vi "saveClampResults-v03.vi"(0 "controls array":refnum<vi>[](array[refnum]), 1 "protocol or memtest":enum16{"protocol", "memtest", "dual"}(ring), 2 "ExpPhase":string, 3 "which clamp":enum16{"VClamp", "IClamp"}(ring), 5 "view profile":waveform(dbl)[](array[waveform]), 9 "rec profile":waveform(dbl)[](array[waveform]), 11 "error in":errorcluster caption="error in (no error)", 12 "metadata to save":T1 {"cell stats"."STD" format="%010.2f"; "cell stats"."Variance" format="%010.2f"; "cell stats"."Rt (MOhms)" format="%010.2f"; "cell stats"."tau (ms)" format="%08.2g"; "cell stats"."Cm (pF)" format="%08.2f"; "cell stats"."Ra (MOhms)" format="%010.2f"; "cell stats"."Rm (MOhms)" format="%010.2f"; "cell stats"."Ihold (pA)" format="%010.2f"}, 14 "Save to (folder dir)":path=path "C:/DATA/8-27-15 save func testing") -> (4 "controls array out":refnum<vi>[](array[refnum]), 15 "error out":errorcluster)   [LabVIEW 2019]
uses:
  autoWC/get_data_from_control_boolean.vi
  wc_protocol_v1.003 Folder/whole_cell_protocol/Controls/cell_stats-v02.ctl
  wc_protocol_v1.003 Folder/whole_cell_protocol/Controls/metadata_to_save.ctl
panel:
  out "rec path out":path
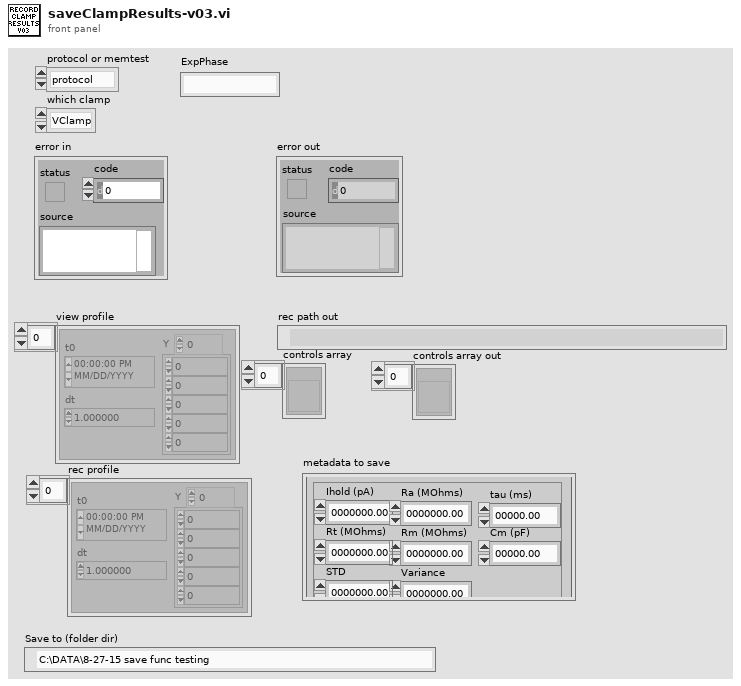
[diagram p1: front panel]
types:
  T1 = typedef "metadata_to_save.ctl" = cluster{"cell stats":T2}
  T2 = typedef "cell_stats-v02.ctl" = cluster{"Ihold (pA)":dbl, "Rm (MOhms)":dbl, "Ra (MOhms)":dbl, "Cm (pF)":dbl, "tau (ms)":dbl, "Rt (MOhms)":dbl, "Variance":dbl, "STD":dbl}
  T3 = enum16{"open", "replace", "create", "open or create", "replace or create", "replace or create with confirmation"}
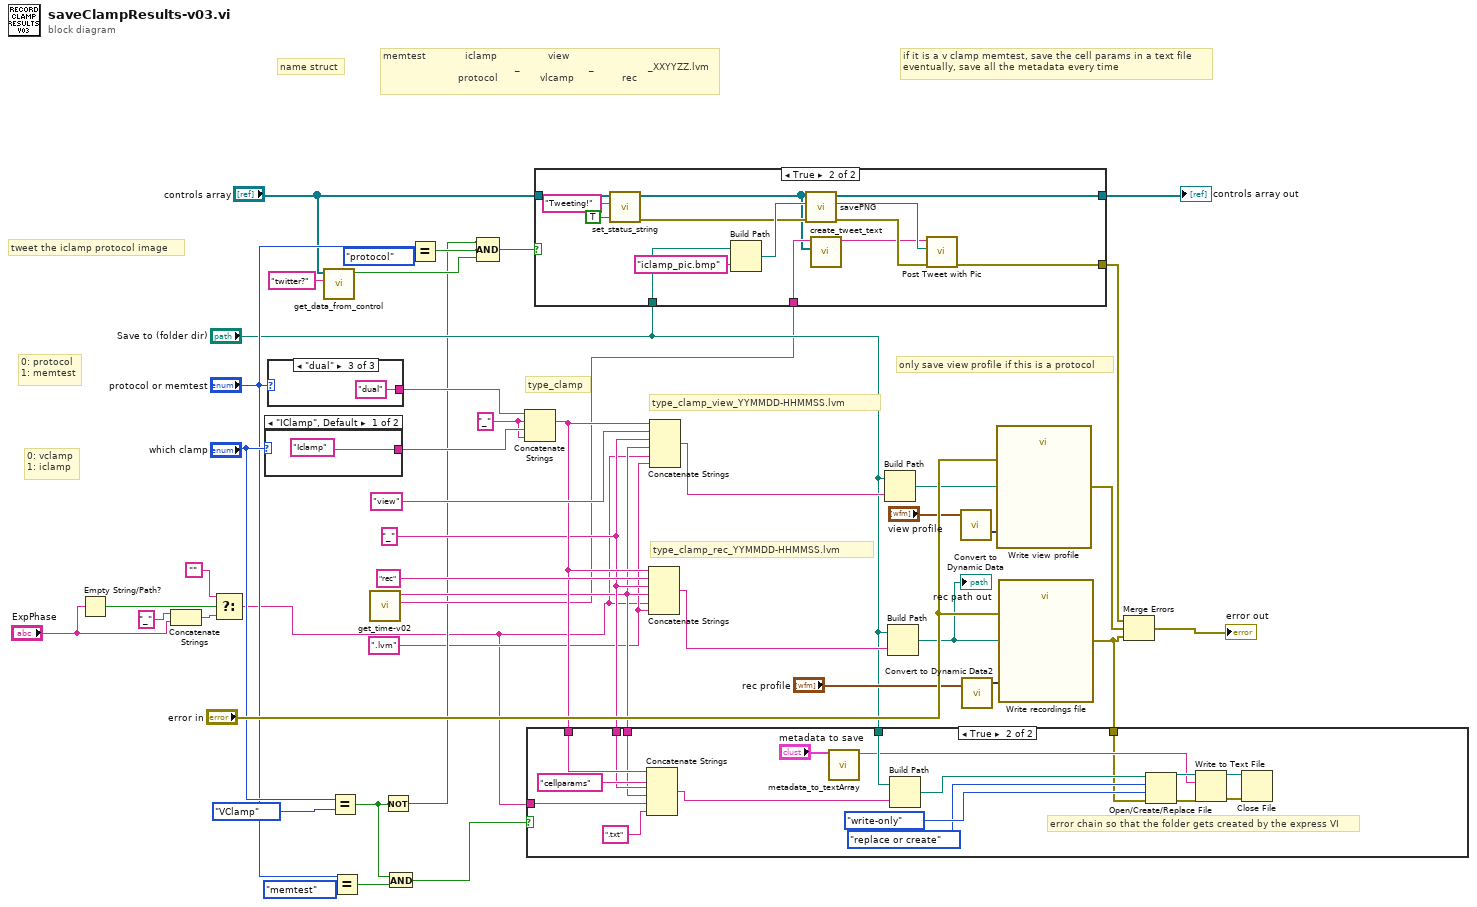
[diagram p0: block diagram]
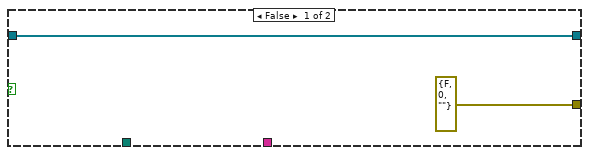
[diagram p2: hidden frame]
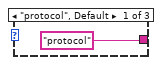
[diagram p4: hidden frame]
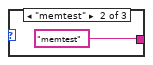
[diagram p5: hidden frame]
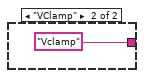
[diagram p6: hidden frame]
diagram:
  w7 = ".lvm" ("name or relative path")
  w24 = "_" ("string")
  w39 = "_" ("string")
  # "tweet the iclamp protocol image"
  # "if it is a v clamp memtest, save the cell params in a text file\neventually, save all the metadata every time"
  # "only save view profile if this is a protocol"
  # "type_clamp_rec_YYMMDD-HHMMSS.lvm"
  # "type_clamp_view_YYMMDD-HHMMSS.lvm"
  # "type_clamp"
  # "name struct"
  # "memtest             iclamp                 view            \n                                            _                       _                  _XXYYZZ.lvm\n                         protocol              vlcamp                rec"
  # "0: protocol\n1: memtest"
  # "0: vclamp\n1: iclamp"
  n1 = Empty String/Path?(string/path="ExpPhase") -> (empty?=w6:bool)
  n2 = Concatenate Strings("_" ("string"), "ExpPhase") -> (w3:string)
  n3 = Select(t="", s=w6, f=w3) -> (s? t:f=w1:string)
  n4 = case shown="\"IClamp\", Default" "which clamp" {
    tunnel: ["Iclamp" "Vclamp"] -> w40
    frame "IClamp", Default {
    }
    frame "VClamp" {
    }
  }
  n5 = case shown="\"dual\"" "protocol or memtest" {
    tunnel: ["protocol" "memtest" "dual"] -> w41
    frame "protocol", Default {
    }
    frame "memtest" {
    }
    frame "dual" {
    }
  }
  n6 = call-poly "get_data_from_control.vi"("control label"="twitter?", "controls array"="controls array") -> ("Boolean"=w14:bool)  [unwired: 8 in, 1 out]
  n7 = Equal?(x="which clamp", y=enum16{"VClamp", "IClamp"}."VClamp") -> (x = y?=w9:bool)
  n8 = Equal?(x="protocol or memtest", y=enum16{"protocol", "memtest"}."memtest") -> (x = y?=w12:bool)
  n9 = call "get_time-v02.vi"() -> ("time output"=w10:string, "pure text output"=w23:string)  [unwired: 10 in]
  n10 = Not(x=w9) -> (.not. x?=w8:bool)
  n11 = And(x=w9, y=w12) -> (x .and. y?=w26:bool)
  n12 = Equal?(x="protocol or memtest", y=enum16{"protocol", "memtest"}."protocol") -> (x = y?=w19:bool)
  n13 = Compound Arithmetic op=AND(w8, w19, w14) -> (w18:bool)
  n14 = Concatenate Strings(w41, w39, w40, w39) -> (w25:string)
  n15 = case shown="True" w18 {
    tunnel: "controls array" -> [w52 w57]
    tunnel: [w52 w62] -> w17
    tunnel: "Save to (folder dir)" -> [_ w66]
    tunnel: [errorcluster {"status"=FALSE, "code"=0, "source"=""} ("error out") w60] -> w11
    tunnel: w10 -> [_ w59]
    frame False {
    }
    frame True {
      n16 = call "set_status_string.vi"("new line?"=TRUE, "status string in"="Tweeting!", "controls array"=w57) -> ("error out"=w56:errorcluster, "controls array out"=w53:refnum<vi>[])  [unwired: 7 in]
      n17 = Build Path(base path=w66, name or relative path="iclamp_pic.bmp") -> (appended path=w65:path)
      n18 = call "savePNG.vi"("error in"=w56, "image path in (.bmp)"=w65, "controls array in"=w53) -> ("error out"=w61:errorcluster, "image path out (.PNG)"=w63:path, "controls array out"=w62:refnum<vi>[])  [unwired: 6 in]
      n19 = call "create_tweet_text.vi"("controls array"=w53, "time string"=w59) -> ("tweet"=w58:string)  [unwired: 9 in]
      n20 = call "Post Tweet with Pic.vi"("error in"=w61, "Picture File (PNG, JPG, GIF)"=w63, "Tweet"=w58) -> ("error out"=w60:errorcluster)  [unwired: 8 in]
    }
  }
  "controls array out" <- w17
  n21 = Concatenate Strings(w25, "rec" ("name or relative path"), w24, w23, w1, w7) -> (w35:string)
  n22 = Concatenate Strings(w25, "view" ("name or relative path"), w24, w23, w1, w7) -> (w36:string)
  n23 = Build Path(base path="Save to (folder dir)", name or relative path=w36) -> (appended path=w31:path)
  n24 = Build Path(base path="Save to (folder dir)", name or relative path=w35) -> (appended path=w33:path)
  "rec path out" <- w33
  n25 = call "Convert to Dynamic Data"("Array of Waveforms"="view profile") -> ("Dynamic Data Type"=w32:dynamicdata)  [unwired: 3 in]
  n26 = call "Convert to Dynamic Data2"("Array of Waveforms"="rec profile") -> ("Dynamic Data Type"=w45:dynamicdata)  [unwired: 3 in]
  n27 = call "Write view profile"("Signals"=w32, "error in (no error)"="error in", "Filename"=w31) -> ("error out"=w43:errorcluster)  [unwired: 14 in, 2 out]
  n28 = call "Write recordings file"("Signals"=w45, "error in (no error)"="error in", "Filename"=w33) -> ("error out"=w22:errorcluster)  [unwired: 14 in, 2 out]
  n29 = case shown="True" w26 {
    tunnel: "Save to (folder dir)" -> [_ w79]
    tunnel: w25 -> [_ w77]
    tunnel: w24 -> [_ w75]
    tunnel: w23 -> [_ w74]
    tunnel: w22 -> [_ w69]
    tunnel: w1 -> [_ w68]
    frame False {
    }
    frame True {
      # "error chain so that the folder gets created by the express VI"
      n30 = Concatenate Strings(w77, "cellparams" ("name or relative path"), w75, w74, w68, ".txt" ("name or relative path")) -> (w78:string)
      n31 = call "metadata_to_textArray.vi"("metadata to save"="metadata to save") -> ("xml string out"=w72:string)  [unwired: 10 in]
      n32 = Build Path(base path=w79, name or relative path=w78) -> (appended path=w80:path)
      n33 = Open/Create/Replace File(file path (use dialog)=w80, error in=w69, operation (0:open)=T3."replace or create", access (0:read/write)=enum16{"read/write", "read-only", "write-only"}."write-only") -> (refnum out=w81:refnum<file>, error out=w83:errorcluster)  [unwired: 2 in, 1 out]
      n34 = Write to Text File(file (use dialog)=w81, text=w72, error in=w83) -> (refnum out=w71:refnum<file>, error out=w82:errorcluster)  [unwired: 1 in, 1 out]
      n35 = Close File(refnum=w71, error in=w82) -> ()  [unwired: 2 out]
    }
  }
  n36 = Merge Errors(w11, w43, w22) -> (→"error out":errorcluster)
